vi "Cryo-Con Get T.vi"(8 "error in (no error)":errorcluster, 10 "Channel":string="A", 11 "VISA Resource Name":refnum<visa-resource-name>) -> (0 "error out":errorcluster, 1 "data string":string, 2 "Temperature":dbl format="%.5f", 3 "VISA Resource Name Out":refnum<visa-resource-name>)   [LabVIEW 2016]
uses:
  <vilib>/Utility/error.llb/Error Cluster From Error Code.vi
  GPIB/VISA  Send Receive.vi
  <vilib>/ErrorRing/Error Ring.xnode
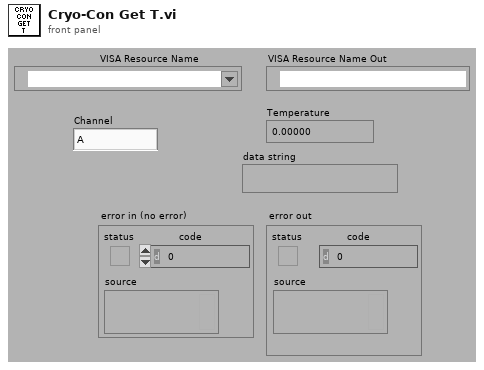
[diagram p1: front panel]
types:
  T1 = enum16{"open", "replace", "create", "open or create", "replace or create", "replace or create with confirmation"}
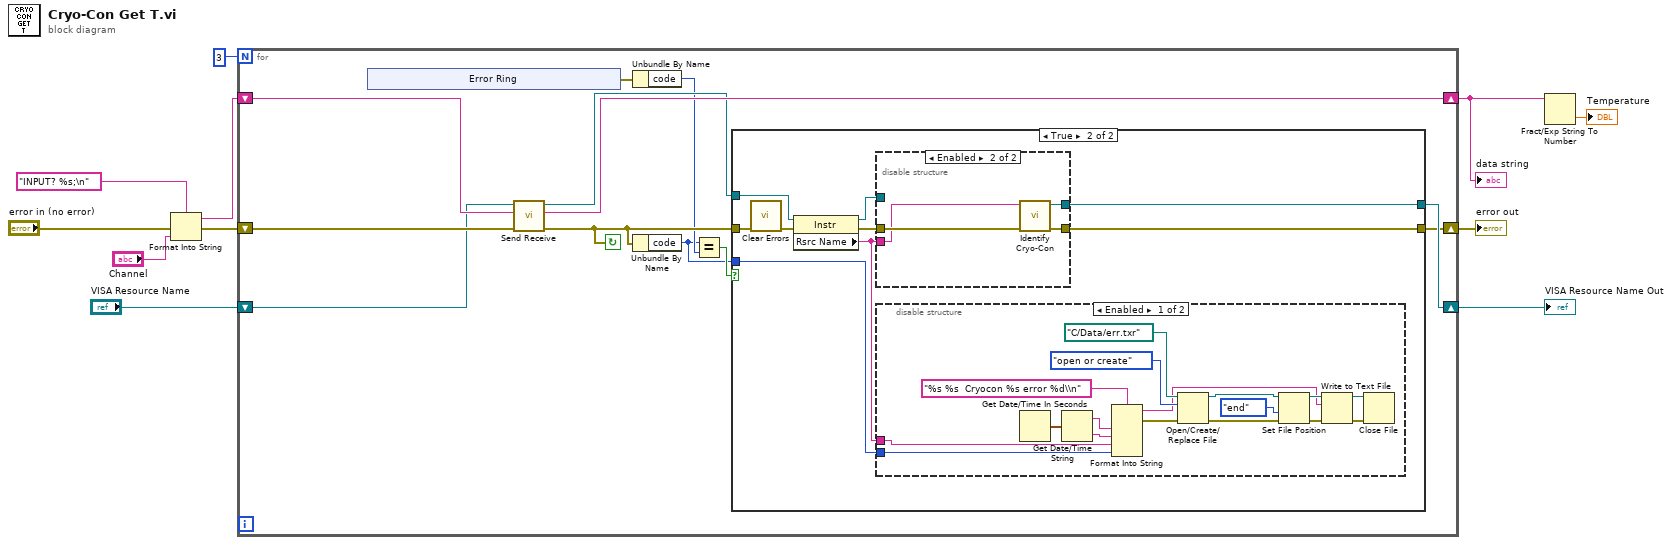
[diagram p0: block diagram]
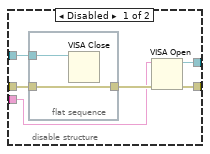
[diagram p3: hidden frame]
diagram:
  n1 = Format Into String(format string="INPUT? %s;\n" ("data string"), error in="error in (no error)", "Channel") -> (resulting string=w5:string, error out=w6:errorcluster)  [unwired: 1 in]
  n2 = for {
    N: 3 -> [_]
    shift-right: [w17] -> w9
    shift-left: "VISA Resource Name" -> [w12]
    shift-right: [w15] -> w11
    shift-left: w6 -> [w23]
    shift-right: [w21] -> w4
    shift-left: w5 -> [w22]
    stop <- w16 continue-if-true
    n3 = xnode "Error Ring"() -> ("error out"=w20:errorcluster)
    n4 = call-poly "Send Receive.vi"("error in (no error)"=w23, "data string in"=w22, "VISA Resource Name"=w12) -> ("error out"=w16:errorcluster, "data string out"=w21:string, "VISA Resource Name Out"=w18:refnum<visa-resource-name>)  [unwired: 6 in]
    n5 = Unbundle By Name(w20) -> ("code"=w14:i32)
    n6 = Unbundle By Name(w16) -> ("code"=w13:i32)
    n7 = Equal?(x=w13, y=w14) -> (x = y?=w19:bool)
    n8 = case shown="True" w19 {
      tunnel: w16 -> [w25 w34]
      tunnel: w18 -> [w24 w31]
      tunnel: [w25 w29] -> w15
      tunnel: [w24 w28] -> w17
      tunnel: w13 -> [_ w26]
      frame False {
      }
      frame True {
        n9 = call <vilib>:"Clear Errors.vi"("error in (no error)"=w34) -> ("error out"=w33:errorcluster)  [unwired: 5 in, 1 out]
        n10 = property class="Instr"(reference=w31, error in=w33) -> (reference out=w32:refnum<visa-resource-name>, error out=w30:errorcluster, "Rsrc Name"=w27:string)
        n11 = disable-structure shown="Enabled" {
          disable-tunnel: w32 -> [w40 _]
          disable-tunnel: w30 -> [w39 w46]
          disable-tunnel: [w37 w44] -> w29
          disable-tunnel: [w36 w43] -> w28
          disable-tunnel: w27 -> [w35 w45]
          frame Disabled {
            n12 = flat-sequence {
              tunnel: w40 -> [w42]
              tunnel: w39 -> [w41]
              tunnel: [w41] -> w38
              frame #0 {
                n13 = VISA Close(VISA resource name=w42) -> ()  [unwired: 1 in, 1 out]
              }
            }
            n14 = VISA Open(error in (no error)=w38, VISA resource name=w35) -> (VISA resource name=w36:refnum<visa-resource-name>, error out=w37:errorcluster)  [unwired: 3 in]
          }
          frame Enabled {
            n15 = call "Identify Cryo-Con.vi"("Error In"=w46, "VISA resource name"=w45) -> ("Error Out"=w44:errorcluster, "VISA resource name out"=w43:refnum<visa-resource-name>)  [unwired: 6 in, 2 out]
          }
        }
        n16 = disable-structure shown="Enabled" {
          disable-tunnel: w27 -> [w50 _]
          disable-tunnel: w26 -> [w49 _]
          frame Enabled {
            n17 = Get Date/Time In Seconds() -> (seconds since 1Jan1904=w53:timestamp)
            n18 = Get Date/Time String(seconds (now)=w53) -> (date string=w52:string, time string=w51:string)  [unwired: 2 in]
            n19 = Format Into String(format string="%s %s  Cryocon %s error %d\\n", w52, w51, w50, w49) -> (resulting string=w48:string, error out=w47:errorcluster)  [unwired: 2 in]
            n20 = Open/Create/Replace File(file path (use dialog)=path "C:/Data/err.txr" ("file (use dialog)"), error in=w47, operation (0:open)=T1."open or create") -> (refnum out=w61:refnum<file>, error out=w58:errorcluster)  [unwired: 3 in, 1 out]
            n21 = Set File Position(refnum=w61, from (0:start)=enum16{"start", "end", "current"}."end", error in=w58) -> (refnum out=w60:refnum<file>, error out=w57:errorcluster)  [unwired: 1 in]
            n22 = Write to Text File(file (use dialog)=w60, text=w48, error in=w57) -> (refnum out=w55:refnum<file>, error out=w56:errorcluster)  [unwired: 1 in, 1 out]
            n23 = Close File(refnum=w55, error in=w56) -> ()  [unwired: 2 out]
          }
          frame Disabled {
          }
        }
      }
    }
  }
  "error out" <- w11
  "data string" <- w4
  "VISA Resource Name Out" <- w9
  n24 = Fract/Exp String To Number(string=w4) -> (number=→"Temperature":dbl)  [unwired: 4 out]
